vi "Sort scan settings.vi"(7 "Scan settings array":T1[](array[typedef]) {"Number of pixels to stabilize \nper substrate" items=["1", "2", "3", "4", "5", "6", "7", "8"]; "Range Options" items=["Auto Range", "100 uA", "1 mA", "10 mA", "100 mA", "1A"]}, 10 "Setting name array":string[](array[string])) -> (0 "Sorted settings array":T1[](array[typedef]) {"Number of pixels to stabilize \nper substrate" items=["1", "2", "3", "4", "5", "6", "7", "8"]; "Range Options" items=["Auto Range", "100 uA", "1 mA", "10 mA", "100 mA", "1A"]}, 3 "Sorted name array":string[](array[string]))   [LabVIEW 2011]
uses:
  Typedefs/Scan settings.ctl
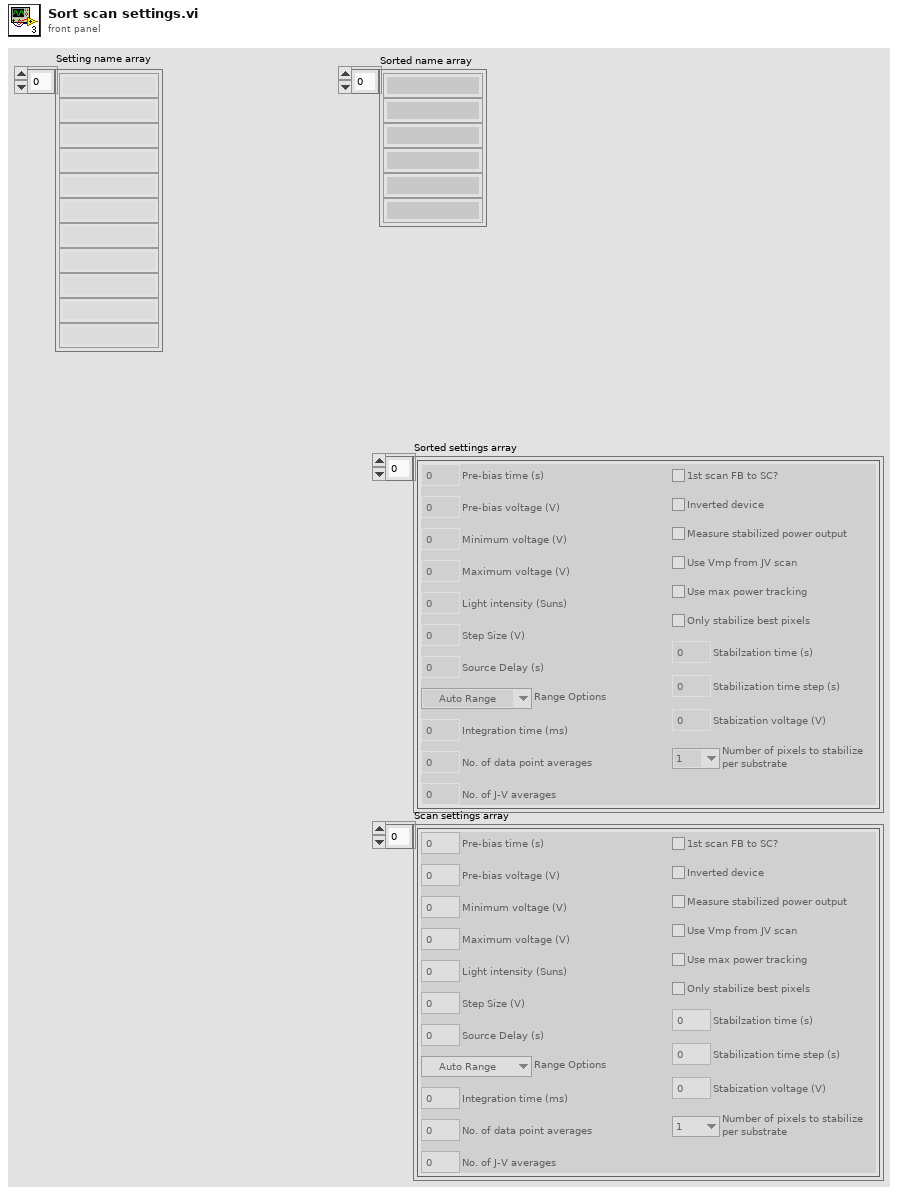
[diagram p1: front panel]
types:
  T1 = typedef "Scan settings.ctl" = cluster{"Light intensity (Suns)":dbl, "Pre-bias time (s)":dbl, "Maximum voltage (V)":dbl, "Minimum voltage (V)":dbl, "Range Options":u16, "1st scan FB to SC?":bool, "Step Size (V)":dbl, "Source Delay (s)":dbl, "Inverted device":bool, "Measure stabilized power output":bool, "Stabilzation time (s)":dbl, "Use Vmp from JV scan":bool, "Stabization voltage (V)":dbl, "Only stabilize best pixels":bool, "Number of pixels to stabilize \nper substrate":u16, "Stabilization time step (s)":dbl, "Use max power tracking":bool, "Pre-bias voltage (V)":dbl, "No. of data point averages":dbl, "No. of J-V averages":dbl, "Integration time (ms)":dbl}
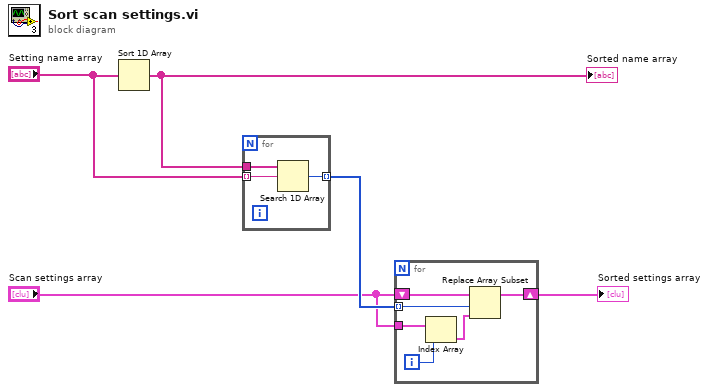
[diagram p0: block diagram]
diagram:
  n1 = Sort 1D Array(array="Setting name array") -> (sorted array=w5:string[])
  "Sorted name array" <- w5
  n2 = for {
    tunnel: w5 -> [w8]
    tunnel: "Setting name array" -> [w7] mode=indexing
    tunnel: [w6] -> w3 mode=indexing
    n3 = Search 1D Array(1D array=w8, element=w7) -> (index of element=w6:i32)  [unwired: 1 in]
  }
  n4 = for {
    shift-right: [w13] -> w2
    shift-left: "Scan settings array" -> [w14]
    tunnel: "Scan settings array" -> [w12]
    tunnel: w3 -> [w10] mode=indexing
    i -> [w9]
    n5 = Index Array(array=w12, index=w9) -> (element=w11:T1)
    n6 = Replace Array Subset(array=w14, new element=w11, index=w10) -> (w13:T1[])
  }
  "Sorted settings array" <- w2
